vi "Get Initial Val.vi"(8 "error in":errorcluster, 9 "IMAGE SAVE FORMAT":u32, 10 "String":string, 11 "gRPC ID In":T1) -> (0 "error out":errorcluster)   [LabVIEW 2026]
uses:
  Automotive-Vision-OOBService_client/Automotive-Vision-OOBService_client.lvlib
  Automotive-Vision-OOBService_client/RPC Messages/hwval_ExportRequest.ctl
  Automotive-Vision-OOBService_client/RPC Messages/hwval_ExportFileType.ctl
  Automotive-Vision-OOBService_client/RPC Messages/hwval_ExportTypeRequest.ctl
  <vilib>/gRPC/LabVIEW gRPC Library/Shared/grpcId.ctl
  <vilib>/gRPC/LabVIEW gRPC Library/grpc-lvsupport-release.lvlib
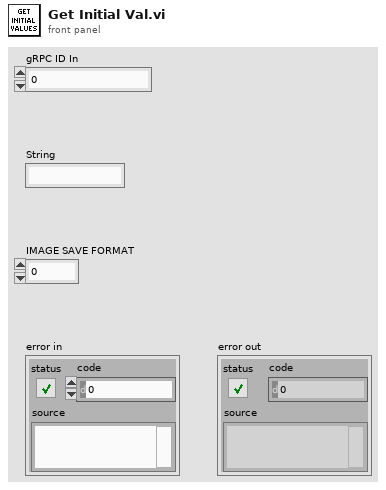
[diagram p1: front panel]
types:
  T1 = typedef "grpc-lvsupport-release.lvlib/grpcId.ctl" = u64
  T2 = typedef "Automotive-Vision-OOBService_client.lvlib/hwval_ExportTypeRequest.ctl" = cluster{"FileType":T3}
  T3 = typedef "Automotive-Vision-OOBService_client.lvlib/hwval_ExportFileType.ctl" = enum32{"EXPORT_PNG", "EXPORT_RAW"}
  T4 = typedef "Automotive-Vision-OOBService_client.lvlib/hwval_ExportRequest.ctl" = cluster{"FilePath":string}
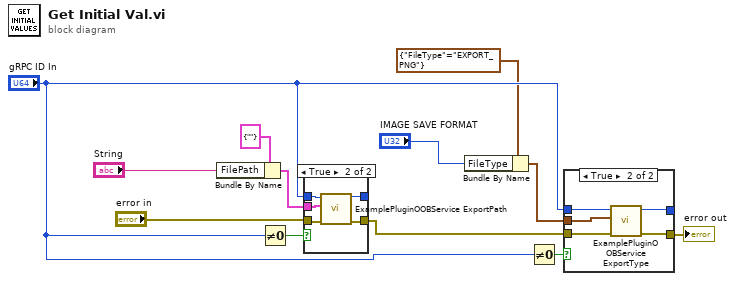
[diagram p0: block diagram]
diagram:
  n1 = Bundle By Name(cluster=T4 {"FilePath"=""} ("Request Data"), "FilePath"="String") -> (w5:T4)
  n2 = Not Equal To 0?(x="gRPC ID In") -> (x != 0?=w2:bool)
  n3 = case shown="True" w2 {
    tunnel: [w14 w18] -> _
    tunnel: [w13 w16] -> w10
    tunnel: "gRPC ID In" -> [w14 w19]
    tunnel: "error in" -> [w13 w17]
    tunnel: w5 -> [_ w15]
    frame False {
    }
    frame True {
      n4 = call "ExamplePluginOOBService ExportPath.vi"("error in"=w17, "Request Data"=w15, "gRPC ID"=w19) -> ("error out"=w16:errorcluster, "gRPC ID out"=w18:T1)  [unwired: 6 in, 1 out]
    }
  }
  n5 = Bundle By Name(cluster=T2 {"FileType"=enum."EXPORT_PNG"} ("Request Data"), "FileType"="IMAGE SAVE FORMAT") -> (w8:T2)
  n6 = Not Equal To 0?(x="gRPC ID In") -> (x != 0?=w6:bool)
  n7 = case shown="True" w6 {
    tunnel: w10 -> [w20 w24]
    tunnel: [w20 w23] -> w1
    tunnel: "gRPC ID In" -> [w21 w25]
    tunnel: [w21 w22] -> _
    tunnel: w8 -> [_ w26]
    frame False {
    }
    frame True {
      n8 = call "ExamplePluginOOBService ExportType.vi"("error in"=w24, "Request Data"=w26, "gRPC ID"=w25) -> ("error out"=w23:errorcluster, "gRPC ID out"=w22:T1)  [unwired: 6 in, 1 out]
    }
  }
  "error out" <- w1
